vi "LCD Custom Character Example.vi"() -> ()   [LabVIEW 2012, in "Phidget LCD.lvlib"]
uses:
  <instrlib>/Phidgets/Phidget LCD/Phidget LCD.lvlib
  <instrlib>/Phidgets/Phidget LCD/Public/LCDStart.vi
  <instrlib>/Phidgets/Phidget LCD/Public/LCDClose.vi
  <instrlib>/Phidgets/Phidget Common/Phidget Common.lvlib
panel:
  in  "Font":u16(ring)=1 items=["FONT_User1"=1, "FONT_User2"=2, "FONT_6x10"=3, "FONT_5x8"=4, "FONT_6x12"=5]
  out "error out":errorcluster
  in  "error in (no error)":errorcluster
  in  "Device Info":T1={"Serial Number"=-1, "Channel"=0, "Port"=0}
  out "Attached?":bool
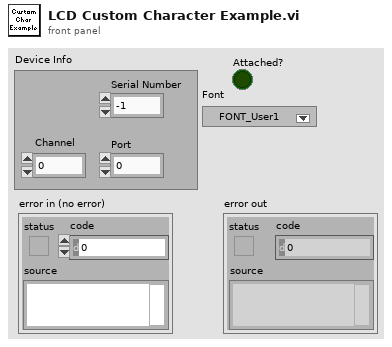
[diagram p1: front panel]
types:
  T1 = cluster{"Serial Number":i32, "Channel":i32, "Port":i32}
  T2 = cluster{bool, bool, bool, bool, bool, bool, bool, bool, bool, bool, bool, bool, bool, bool, bool, bool, bool, bool, bool, bool, bool, bool, bool, bool, bool, bool, bool, bool, bool, bool, bool, bool, bool, bool, bool, bool, bool, bool, bool, bool}
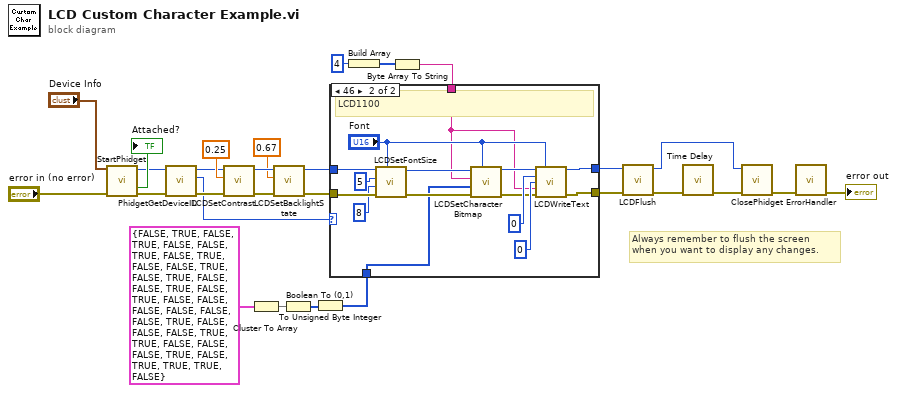
[diagram p0: block diagram]
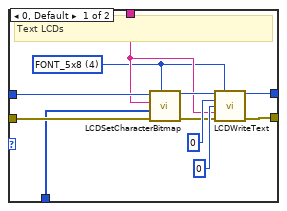
[diagram p2: hidden frame]
diagram:
  # "Always remember to flush the screen\nwhen you want to display any changes."
  n1 = call-poly <instrlib>:"StartPhidget.vi"("Device Info"="Device Info", "error in (no error)"="error in (no error)") -> ("Phidget ID"=w3:u64, "Attached?"=→"Attached?":bool, "error out"=w2:errorcluster)  [unwired: 10 in, 1 out]
  n2 = call <instrlib>:"PhidgetGetDeviceID.vi"("error in (no error)"=w2, "Device In"=w3) -> ("error out"=w5:errorcluster, "Devie IDs"=w1:u32, "Device Out"=w4:u64)  [unwired: 6 in]
  n3 = call <instrlib>:"LCDSetContrast.vi"("error in (no error)"=w5, "Contrast"=0.25, "Device In"=w4) -> ("error out"=w22:errorcluster, "Device Out"=w21:u64)  [unwired: 6 in]
  n4 = Cluster To Array(cluster=T2 {FALSE, TRUE, FALSE, TRUE, FALSE, FALSE, TRUE, FALSE, TRUE, FALSE, FALSE, TRUE, FALSE, TRUE, FALSE, FALSE, TRUE, FALSE, TRUE, FALSE, FALSE, FALSE, FALSE, FALSE, FALSE, TRUE, FALSE, FALSE, FALSE, TRUE, TRUE, FALSE, FALSE, FALSE, TRUE, FALSE, TRUE, TRUE, TRUE, FALSE}) -> (array=w13:bool[])
  n5 = call <instrlib>:"LCDSetBacklightState.vi"("error in (no error)"=w22, "Backlight"=0.67 ("Contrast"), "Device In"=w21) -> ("error out"=w17:errorcluster, "Device Out"=w18:u64)  [unwired: 6 in]
  n6 = Boolean To (0,1)(Boolean=w13) -> (0, 1=w7:i16[])
  n7 = To Unsigned Byte Integer(number=w7) -> (unsigned 8bit integer=w6:u8[])
  n8 = Build Array(u8 4 ("Character")) -> (w15:u8[])
  n9 = Byte Array To String(unsigned byte array=w15) -> (string=w10:string)
  n10 = case shown="46" w1 {
    tunnel: w18 -> [w39 w48]
    tunnel: w17 -> [w38 w47]
    tunnel: [w35 w52] -> w12
    tunnel: [w34 w51] -> w11
    tunnel: w10 -> [w30 w41]
    tunnel: w6 -> [w31 w40]
    frame 0, Default {
      w29 = u16 4 items=["FONT_User1"=1, "FONT_User2"=2, "FONT_6x10"=3, "FONT_5x8"=4, "FONT_6x12"=5] ("Font")
      # "Text LCDs"
      n11 = call <instrlib>:"LCDSetCharacterBitmap.vi"("Font"=w29, "error in (no error)"=w38, "Bitmap"=w31, "Character"=w30, "Device In"=w39) -> ("error out"=w32:errorcluster, "Device Out"=w33:u64)  [unwired: 5 in]
      n12 = call <instrlib>:"LCDWriteText.vi"("Device In"=w33, "Font"=w29, "xpos"=0, "ypos"=0, "Text"=w30, "error in (no error)"=w32) -> ("Device Out"=w35:u64, "error out"=w34:errorcluster)  [unwired: 8 in]
    }
    frame 70 {
      # "LCD1100"
      n13 = call <instrlib>:"LCDSetFontSize.vi"("Font"="Font", "error in (no error)"=w47, "height"=8, "width"=5, "Device In"=w48) -> ("error out"=w42:errorcluster, "Device Out"=w43:u64)  [unwired: 5 in]
      n14 = call <instrlib>:"LCDSetCharacterBitmap.vi"("Font"="Font", "error in (no error)"=w42, "Bitmap"=w40, "Character"=w41, "Device In"=w43) -> ("error out"=w49:errorcluster, "Device Out"=w50:u64)  [unwired: 5 in]
      n15 = call <instrlib>:"LCDWriteText.vi"("Device In"=w50, "Font"="Font", "xpos"=0, "ypos"=0, "Text"=w41, "error in (no error)"=w49) -> ("Device Out"=w52:u64, "error out"=w51:errorcluster)  [unwired: 8 in]
    }
  }
  n16 = call <instrlib>:"LCDFlush.vi"("error in (no error)"=w11, "Device In"=w12) -> ("error out"=w9:errorcluster, "Device Out"=w23:u64)  [unwired: 7 in]
  n17 = call "Time Delay"("error in (no error)"=w9) -> ("error out"=w8:errorcluster)  [unwired: 10 in]
  n18 = call-poly <instrlib>:"ClosePhidget.vi"("error in"=w8, "Device In"=w23) -> ("error out"=w25:errorcluster)  [unwired: 9 in]
  n19 = call <instrlib>:"ErrorHandler.vi"("error in"=w25) -> ("error out"=→"error out":errorcluster)  [unwired: 9 in, 1 out]
